vi "TEST_L0_SUMnADDS_(2ND)_NEW.vi"(7 "Serial Number":string="testFile", 8 "error in (no error)":errorcluster, 11 "Instrument VISA in":T1={"AWG VISA"="generadorpulsos", "Oscilloscope  VISA "="Oscilloscope", "Integration Board IP"="172.16.7.43", "connection ID"=refnum, "report out"=refnum, "report file path"=path "C:/Documents and Settings/CTA_LAB01/Desktop/L0_Asic/L0 Asic Test Data"}) -> (0 "error out":errorcluster, 3 "Instrument VISA out":T1={"AWG VISA"="generadorpulsos", "Oscilloscope  VISA "="Oscilloscope", "Integration Board IP"="172.16.7.43", "connection ID"=refnum, "report out"=refnum, "report file path"=path "C:/Documents and Settings/CTA_LAB01/Desktop/L0_Asic/L0 Asic Test Data"})   [LabVIEW 2009]
uses:
  <vilib>/Utility/NIReport.llb/NI_report.lvclass
  <vilib>/Utility/NIReport.llb/HTML/NI_HTML.lvclass
  Sum_Abrilader/L0_Sum_Adder Folder/C/Program Files/National Instruments/LabVIEW 2012/instr.lib/Agilent 8000 Series/Public/Configure/Configure Math (Binary Operation).vi
  <instrlib>/Agilent 8000 Series/Public/Data/Low Level/Fetch Measurement (More).vi
  <instrlib>/Agilent 8000 Series/Agilent 8000 Series.lvlib
panel:
  in  "Channels \nCombinations":i32[](array[numeric])=[3, 12, 48, 96, 7, 28, 112, 15, 120, 31, 124, 63, 126, 127]
  in  "Voltages":dbl[](array[numeric])=[0.05, 0.1, 0.2, 0.5, 0.8]
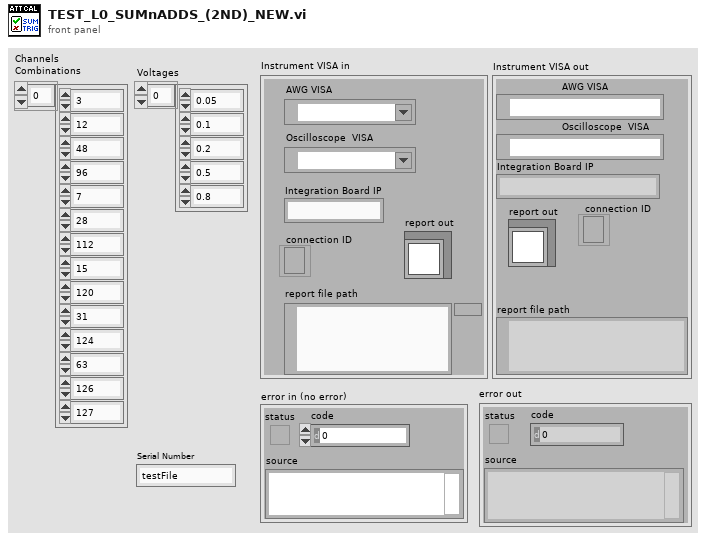
[diagram p1: front panel]
types:
  T1 = cluster{"AWG VISA":refnum<visa-resource-name>, "Oscilloscope  VISA ":refnum<visa-resource-name>, "Integration Board IP":string, "connection ID":refnum<k5>, "report out":refnum<class "NI_report.lvclass">, "report file path":path}
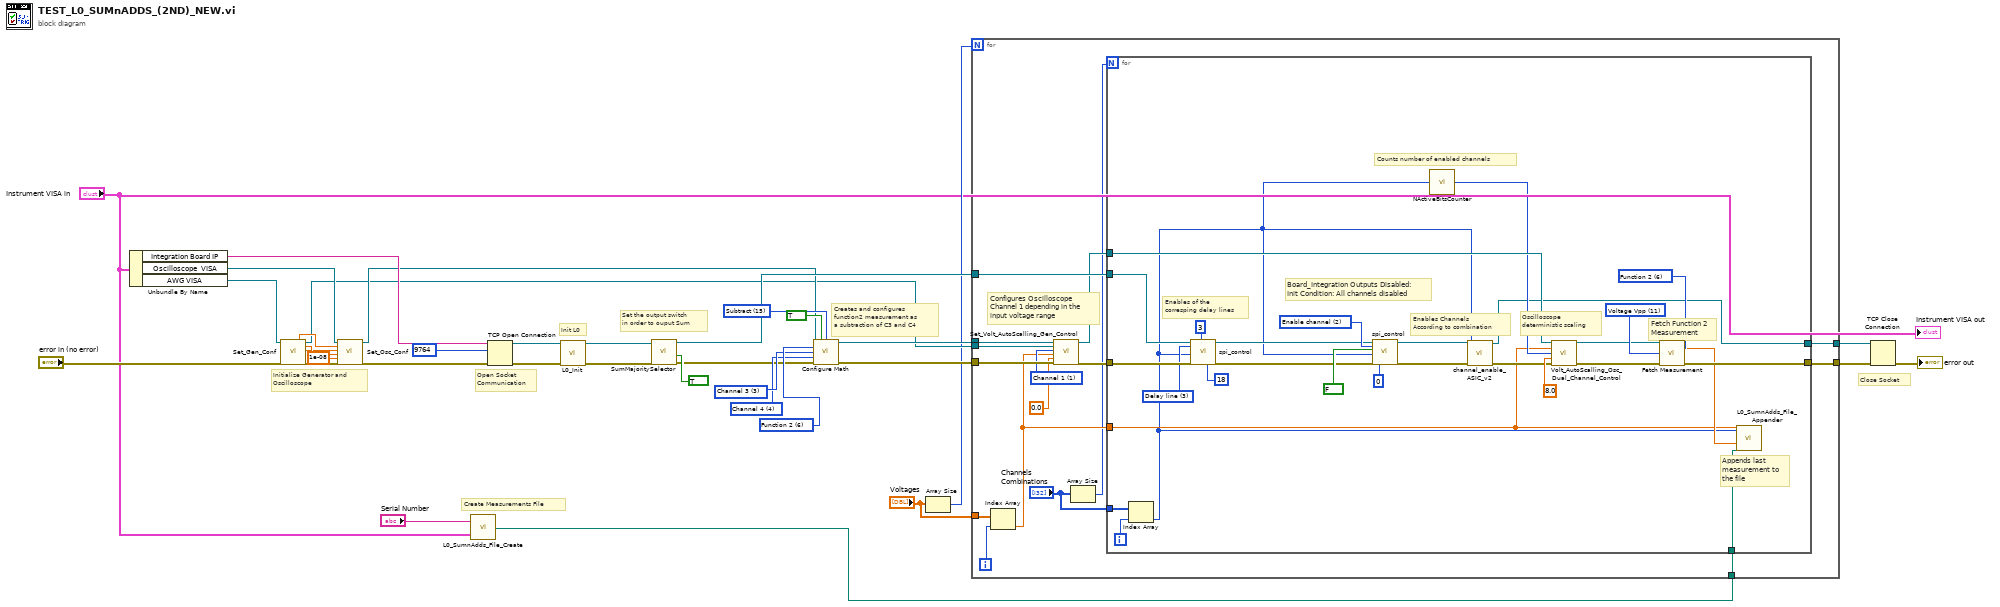
[diagram p0: block diagram]
diagram:
  w32 = u16 6 items=["Function 1"=5, "Function 2"=6, "Function 3"=7, "Function 4"=8] ("Math Channel (5: Function 1)")
  w33 = u16 15 items=["Add"=12, "Divide"=13, "Multiply"=14, "Subtract"=15, "Common Mode"=16, "Versus"=17] ("Math Operation (12: Add)")
  w31 = 3 items=["Channel 1"=1, "Channel 2"=2, "Channel 3"=3, "Channel 4"=4] ("Channel (1: Channel 1)")
  w30 = 4 items=["Channel 1"=1, "Channel 2"=2, "Channel 3"=3, "Channel 4"=4] ("Channel (1: Channel 1)")
  # "Close Socket"
  # "Create Measurements File"
  # "Initialize Generator and \nOscilloscope"
  # "Init L0"
  # "Creates and configures\nfunction2 measurement as\na subtraction of C3 and C4"
  # "Set the output switch\nin order to ouput Sum"
  # "Open Socket\nCommunication"
  n1 = Unbundle By Name("Instrument VISA in") -> ("Integration Board IP"=w25:string, "Oscilloscope  VISA"=w12:refnum<visa-resource-name>, "AWG VISA"=w13:refnum<visa-resource-name>)
  n2 = call "Set_Gen_Conf.vi"("AWG VISA"=w13, "error in (no error)"="error in (no error)") -> ("Amplitude 1 OUT"=w18:dbl, "VISA resource name out"=w10:refnum<visa-resource-name>, "Pulse Width in seconds 1 OUT"=w17:dbl, "Trigger Level 1"=w16:dbl, "error out"=w19:errorcluster)  [unwired: 10 in, 3 out]
  n3 = call "Set_Osc_Conf.vi"("VISA resource name"=w12, "Amplitude IN"=w18, "Trigger Level IN"=w16, "Pulse Width in seconds IN"=w17, "Position 1"=1e-08, "error in (no error)"=w19) -> ("VISA resource name out"=w11:refnum<visa-resource-name>, "error out"=w14:errorcluster)  [unwired: 12 in]
  n4 = call "L0_SumnAdds_File_Create.vi"("input cluster"="Instrument VISA in", "Serial Number"="Serial Number") -> ("appended path"=w4:path)
  n5 = TCP Open Connection(address=w25, remote port or service name=u16 9764, error in (no error)=w14) -> (connection ID=w24:refnum<k5>, error out=w23:errorcluster)  [unwired: 2 in]
  n6 = call "L0_Init.vi"("error in"=w23, "connection ID in"=w24) -> ("error out"=w21:errorcluster, "connection ID out"=w22:refnum<k5>)  [unwired: 8 in]
  n7 = call "SumMajoritySelector.vi"("On Sum\nOff Majority"=TRUE ("On Sum\nOff Majority"), "error in (no error)"=w21, "connection ID"=w22) -> ("error out"=w26:errorcluster, "connection ID out"=w27:refnum<k5>)  [unwired: 5 in]
  n8 = call-poly "Configure Math.vi"("VISA resource name"=w11, "Enable Math Channel (T:Enable)"=TRUE, "Math Operation (12: Add)"=w33, "Math Channel (5: Function 1)"=w32, "Math Operand (1: Channel 1)"=w31, "Math Operand (2: Channel 2)"=w30, "error in (no error)"=w26) -> ("VISA resource name out"=w20:refnum<visa-resource-name>, "error out"=w29:errorcluster)  [unwired: 7 in]
  n9 = Array Size(array="Voltages") -> (size(s)=w8:i32)
  n10 = for {
    N: w8 -> [_]
    tunnel: w29 -> [w51]
    tunnel: w27 -> [w50]
    tunnel: [w49] -> w3
    tunnel: w20 -> [w48]
    tunnel: w10 -> [w47]
    tunnel: "Voltages" -> [w42]
    tunnel: w4 -> [w37]
    tunnel: [w36] -> w1
    i -> [w41]
    w46 = 1 items=["Channel 1"=1, "Channel 2"=2, "Channel 3"=3, "Channel 4"=4] ("Channel")
    # "Configures Oscilloscope\nChannel 1 depending in the \ninput voltage range"
    n11 = Index Array(array=w42, index=w41) -> (element=w40:dbl)
    n12 = call "Set_Volt_AutoScalling_Gen_Control.vi"("VISA Oscilloscope"=w48, "VISA Generator"=w47, "Channel"=w46, "Amplitude"=w40, "DC Offset"=0.0, "error in (no error)"=w51) -> ("VISA Oscilloscope"=w43:refnum<visa-resource-name>, "error out"=w44:errorcluster)  [unwired: 11 in, 1 out]
    n13 = Array Size(array="Channels \nCombinations") -> (size(s)=w38:i32)
    n14 = for {
      N: w38 -> [_]
      tunnel: w50 -> [w79]
      tunnel: [w58] -> w49
      tunnel: w44 -> [w78]
      tunnel: w43 -> [w77]
      tunnel: w40 -> [w54]
      tunnel: "Channels \nCombinations" -> [w63]
      tunnel: w37 -> [w55]
      tunnel: [w52] -> w36
      i -> [w62]
      w61 = 11 items=["Rise Time", "Fall Time", "Frequency", "Period", "Voltage RMS(AC)", "Voltage RMS(DC)", "Voltage RMS (AC,cycle)", "Voltage RMS (DC,cycle)", "Voltage Max", "Voltage Min", "Voltage Middle", "Voltage Vpp", "Voltage High", "Voltage Low", "Voltage Average", "Voltage Average (cycle)", "Width Negative", "Width Positive", "Duty Cycle Positive", "Amplitude", "Overshoot", "Preshoot", "Voltage Base", "Voltage Upper", "Time Max", "Time Min", "Color Grade Crossing", "Color Grade Eye Width", "Color Grade Eye Height", "Color Grade Eye Q-Factory", "Color Grade Eye Duty Cycle Distortion(Percent)", "Color Grade Eye Duty Cycle Distortion(Time)", "Color Grade Eye Jitter(PP)", "Color Grade Eye Width(RMS)", "Cycle-cycle Duty Jitter(Rising)", "Cycle-cycle Duty Jitter(Falling)", "Cycle-cycle Jitter(Rising)", "Cycle-cycle Jitter(Falling)", "Cycle-cycle - Width", "Cycle-cycle + Width", "Date Rate", "Unit Interval", "FFT Delta Frequency", "FFT Delta Magnitude", "FFT Frequency", "FFT Magnitude", "Slew Rate", "Area (Entire Display)", "Area(Single Cycle)", "Duty Cycle (Rising)", "Duty Cycle (Falling)"] ("Measurement Function (0: Rise Time)")
      w60 = 6 items=["Channel 1"=1, "Channel 2"=2, "Channel 3"=3, "Channel 4"=4, "Function 1"=5, "Function 2"=6, "Function 3"=7, "Function 4"=8, "Memory 1"=9, "Memory 2"=10, "Memory 3"=11, "Memory 4"=12] ("Channel (1: Channel 1)")
      w70 = u16 2 items=["Attenuation", "Clipping", "Enable channel", "Delay line", "ASIC"] ("Device")
      w73 = u16 3 items=["Attenuation", "Clipping", "Enable channel", "Delay line", "ASIC"] ("Device")
      # "Counts number of enabled channels"
      # "Enables Channels\nAccording to combination"
      # "Fetch Function 2\nMeasurement"
      # "Appends last\nmeasurement to\nthe file"
      # "Enables of the\ncorresping delay lines"
      # "Board_Integration Outputs Disabled:\nInit Condition: All channels disabled"
      # "Oscilloscope \ndeterministic scaling"
      n15 = Index Array(array=w63, index=w62) -> (element=w53:i32)
      n16 = call "spi_control.vi"("connection ID"=w79, "Device"=w73, "Data"=w53, "Register or channel"=18, "error out 3"=w78, "chip delay"=3) -> ("connection ID out"=w68:refnum<k5>, "error out 2"=w67:errorcluster)  [unwired: 6 in, 6 out]
      n17 = call "spi_control.vi"("connection ID"=w68, "Device"=w70, "Read/#write"=FALSE, "Data"=w53, "error out 3"=w67, "Id in"=0) -> ("connection ID out"=w66:refnum<k5>, "error out 2"=w65:errorcluster)  [unwired: 6 in, 6 out]
      n18 = call "NActiveBitsCounter.vi"("Input Number"=w53) -> ("N High Bits"=w64:i32)
      n19 = call "channel_enable_ASIC_v2.vi"("error in"=w65, "Channel Combination"=w53, "Connection ID in"=w66) -> ("error out"=w72:errorcluster, "Connection ID out"=w52:refnum<k5>)  [unwired: 7 in]
      n20 = call "Volt_AutoScalling_Osc_Dual_Channel_Control.vi"("VISA Oscilloscope"=w77, "Voltage In"=w54, "N Channels"=w64, "Offset Divider"=8.0, "error in"=w72) -> ("VISA resource name out"=w57:refnum<visa-resource-name>, "error out"=w59:errorcluster)  [unwired: 9 in]
      n21 = call-poly <instrlib>:"Fetch Measurement.vi"("VISA resource name"=w57, "Channel (1: Channel 1)"=w60, "Measurement Function (0: Rise Time)"=w61, "error in (no error)"=w59) -> ("Measurement"=w56:dbl, "error out"=w58:errorcluster)  [unwired: 9 in, 1 out]
      n22 = call "L0_SumnAdds_File_Appender.vi"("Vin"=w54, "CH"=w53, "Vmeas"=w56, "file path (dialog if empty)"=w55) -> ()  [unwired: 24 in]
    }
  }
  n23 = TCP Close Connection(connection ID=w1, error in (no error)=w3) -> (error out=→"error out":errorcluster)  [unwired: 1 in, 1 out]
  "Instrument VISA out" <- "Instrument VISA in"
